vi "Put Object from RAW data.vi"(4 "Region":T1, 7 "Request Parameters":T3={"Content Type"="binary/octet-stream", "ACL"=enum."private", "Storage Class"=enum."STANDARD", "User Metadata"=[], "Content MD5"=""}, 8 "error in (no error)":errorcluster, 9 "Bucket":string, 10 "Object Path":string, 11 "Data":string) -> (0 "error out":errorcluster, 3 "PutObjectResult":T2)   [LabVIEW 2015, in "LV Interface for Amazon S3.lvlib"]
doc: "This operation <B>adds an object to a bucket</B>. You <B>must have WRITE permissions on a bucket</B> to add an object to it. Amazon S3 <B>never adds partial objects</B>; if you receive no error response, Amazon S3 added the entire object to the bucket. Amazon S3 is a distributed system. If Amazon S3 receives multiple write requests for the same object simultaneously, all but the last object written will be overwritten. Amazon S3 does not provide object locking; if you need this, make sure to build it into your application layer or use versioning instead."
uses:
  LV Interface for Amazon S3.lvlib
  Typedefs/AMZ_S3_API_PUT Object Request Parameters.ctl
  Typedefs/AMZ_S3_ACL.ctl
  Typedefs/AMZ_S3_Storage Class.ctl
  Typedefs/AMZ_S3_Object Metadata.ctl
  Typedefs/AMZ_S3_API_PUTObjectResult.ctl
  Typedefs/AMZ_S3_LocationConstraint.ctl
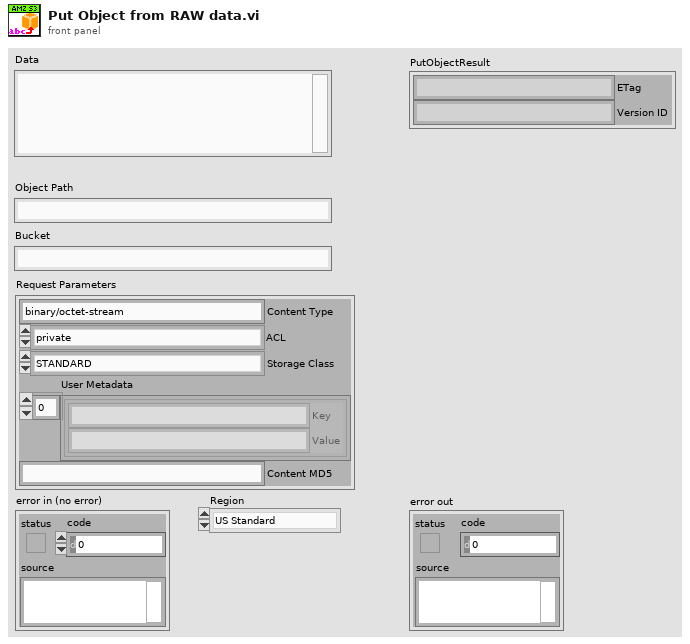
[diagram p1: front panel]
types:
  T1 = typedef "LV Interface for Amazon S3.lvlib/AMZ_S3_LocationConstraint.ctl" = enum16{"US Standard", "us-east-2", "us-west-1", "us-west-2", "ap-northeast-1", "ap-northeast-2", "ap-southeast-1", "ap-southeast-2", "ca-central-1", "eu-central-1", "eu-west-1", "eu-west-2", "sa-east-1"}
  T2 = typedef "LV Interface for Amazon S3.lvlib/AMZ_S3_API_PUTObjectResult.ctl" = cluster{"ETag":string, "Version ID":string}
  T3 = typedef "LV Interface for Amazon S3.lvlib/AMZ_S3_API_PUT Object Request Parameters.ctl" = cluster{"Content Type":string, "ACL":T4, "Storage Class":T5, "User Metadata":T6[], "Content MD5":string}
  T4 = typedef "LV Interface for Amazon S3.lvlib/AMZ_S3_ACL.ctl" = enum16{"private", "public-read", "public-read-write", "aws-exec-read", "authenticated-read", "bucket-owner-read", "bucket-owner-full-control"}
  T5 = typedef "LV Interface for Amazon S3.lvlib/AMZ_S3_Storage Class.ctl" = enum16{"STANDARD", "REDUCED_REDUNDANCY"}
  T6 = typedef "LV Interface for Amazon S3.lvlib/AMZ_S3_Object Metadata.ctl" = cluster{"Key":string, "Value":string}
  T7 = typedef "LV Interface for Amazon S3.lvlib/AMZ_S3_HTTP Header-Value pair.ctl" = cluster{"Header":string, "Value":string}
  T8 = typedef "LV Interface for Amazon S3.lvlib/AMZ_S3_Call Results.ctl" = enum16{"Success", "UndefinedError", "AccessDenied", "AccountProblem", "AmbiguousGrantByEmailAddress", "BadDigest", "BucketAlreadyExists", "BucketAlreadyOwnedByYou", "BucketNotEmpty", "CredentialsNotSupported", "CrossLocationLoggingProhibited", "EntityTooSmall", "EntityTooLarge", "ExpiredToken", "IllegalVersioningConfigurationException", "IncompleteBody", "IncorrectNumberOfFilesInPostRequest", "InlineDataTooLarge", "InternalError", "InvalidAccessKeyId", "InvalidAddressingHeader", "InvalidArgument", "InvalidBucketName", "InvalidDigest", "InvalidLocationConstraint", "InvalidPart", "InvalidPartOrder", "InvalidPayer", "InvalidPolicyDocument", "InvalidRange", "InvalidSecurity", "InvalidSOAPRequest", "InvalidStorageClass", "InvalidTargetBucketForLogging", "InvalidToken", "InvalidURI", "KeyTooLong", "MalformedACLError", "MalformedPOSTRequest", "MalformedXML", "MaxMessageLengthExceeded", "MaxPostPreDataLengthExceededError", "MetadataTooLarge", "MethodNotAllowed", "MissingAttachment", "MissingContentLength", "MissingRequestBodyError", "MissingSecurityElement", "MissingSecurityHeader", "NoLoggingStatusForKey", "NoSuchBucket", "NoSuchKey", "NoSuchUpload", "NoSuchVersion", "NotImplemented", "NotSignedUp", "OperationAborted", "PermanentRedirect", "PreconditionFailed", "Redirect", "RequestIsNotMultiPartContent", "RequestTimeout", "RequestTimeTooSkewed", "RequestTorrentOfBucketError", "SignatureDoesNotMatch", "SlowDown", "TemporaryRedirect", "TokenRefreshRequired", "TooManyBuckets", "UnexpectedContent", "UnresolvableGrantByEmailAddress", "UserKeyMustBeSpecified", "LabVIEWError"}
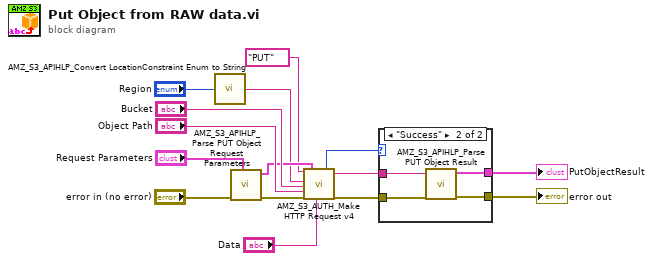
[diagram p0: block diagram]
diagram:
  n1 = call "AMZ_S3_APIHLP_Convert LocationConstraint Enum to String.vi"("Location"="Region") -> ("Location String"=w1:string)  [unwired: 4 in]
  n2 = call "AMZ_S3_APIHLP_Parse PUT Object Request Parameters.vi"("PUT Object Request Parameters"="Request Parameters", "error in (no error)"="error in (no error)") -> ("error out"=w11:errorcluster, "HTTP Headers"=w4:T7[])  [unwired: 8 in]
  n3 = call "AMZ_S3_AUTH_Make HTTP Request v4.vi"("HTTP-Verb"="PUT", "Region"=w1, "Bucket"="Bucket", "Object Key"="Object Path", "error in"=w11, "request headers"=w4, "request body"="Data") -> ("Call Result"=w8:T8, "response headers"=w9:string, "error out"=w10:errorcluster)  [unwired: 9 in, 1 out]
  n4 = case shown="\"Success\"" w8 {
    tunnel: w10 -> [w16 w20]
    tunnel: w9 -> [_ w19]
    tunnel: [_ w18] -> w12
    tunnel: [w16 w17] -> w13
    frame Default {
    }
    frame "Success" {
      n5 = call "AMZ_S3_APIHLP_Parse PUT Object Result.vi"("error in (no error)"=w20, "Response header"=w19) -> ("error out"=w17:errorcluster, "PutObjectResult"=w18:T2)  [unwired: 8 in]
    }
  }
  "error out" <- w13
  "PutObjectResult" <- w12
